vi "Get Interface Count.vi"(8 "error in (no error)":errorcluster) -> (0 "error out":errorcluster, 3 "count":i32)   [LabVIEW 2018, in "lvwpcap.lvlib"]
doc: "This VI outputs the number of active ethernet interfaces in your computer."
uses:
  lvwpcap.lvlib
  lvwpcap.dll
panel:
  # "Select Help»Show Context Help and move the cursor over the VI icon to display help for this VI."
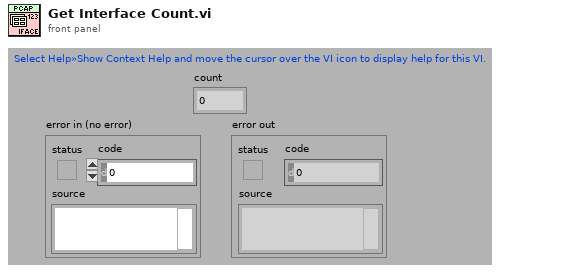
[diagram p1: front panel]
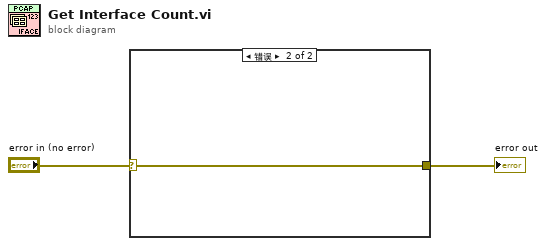
[diagram p0: block diagram]
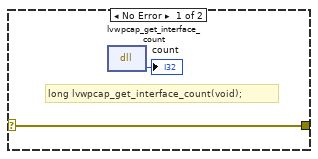
[diagram p2: hidden frame]
diagram:
  n1 = case shown="错误" "error in (no error)" {
    selector: "error in (no error)" -> [w3 w5]
    tunnel: [w3 w5] -> w1
    frame No Error {
      # "long lvwpcap_get_interface_count(void);"
      n2 = dll-call lib="PTH2:abs G论坛资料packet_sniffer_projectlvwpcap.dll" fn="lvwpcap_get_interface_count"() -> (→"count":i32)  [unwired: 3 in, 2 out]
    }
    frame Error {
    }
  }
  "error out" <- w1
